vi "Create String2.vi"(4 "Heart Rate":u32, 6 "Cadence":dbl, 7 "String in":string, 8 "Torque Motor":dbl, 9 "Power":dbl, 10 "Torque Rider":dbl, 11 "t0":timestamp) -> (3 "String out":string)   [LabVIEW 2013]
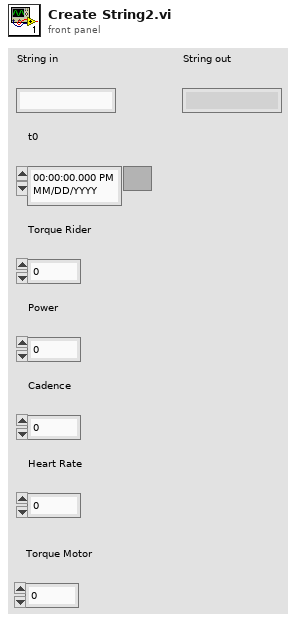
[diagram p1: front panel]
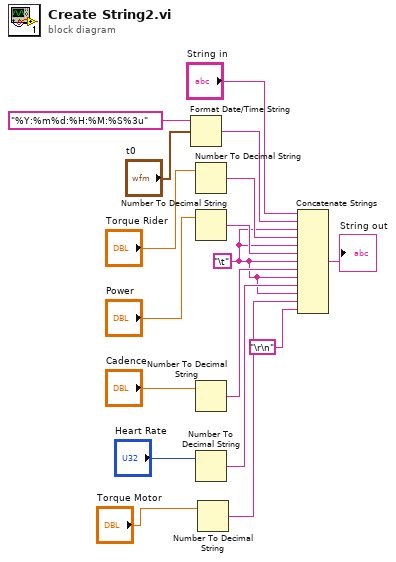
[diagram p0: block diagram]
diagram:
  w3 = "\t"
  n1 = Format Date/Time String(time format string (%c)="%Y:%m%d:%H:%M:%S%3u", seconds (now)="t0") -> (date/time string=w8:string)  [unwired: 1 in]
  n2 = Number To Decimal String(number="Torque Rider") -> (decimal integer string=w11:string)  [unwired: 1 in]
  n3 = Number To Decimal String(number="Power") -> (decimal integer string=w12:string)  [unwired: 1 in]
  n4 = Number To Decimal String(number="Cadence") -> (decimal integer string=w13:string)  [unwired: 1 in]
  n5 = Number To Decimal String(number="Heart Rate") -> (decimal integer string=w17:string)  [unwired: 1 in]
  n6 = Number To Decimal String(number="Torque Motor") -> (decimal integer string=w2:string)  [unwired: 1 in]
  n7 = Concatenate Strings("String in", w8, w3, w11, w3, w12, w3, w13, w3, w17, w3, w2, "\r\n") -> (→"String out":string)
